vi "error_channelIndex.vi"() -> (0 "error out":errorcluster)   [LabVIEW 2020, in "NI_ExcelFile.lvlib"]
uses:
  <vilib>/express/express shared/NI_ExcelFile/NI_ExcelFile.lvlib
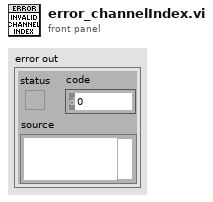
[diagram p1: front panel]
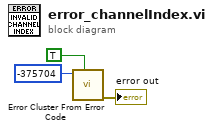
[diagram p0: block diagram]
diagram:
  n1 = call <vilib>:"Error Cluster From Error Code.vi"("show call chain? (False)"=TRUE, "error code (0)"=-375704 ("code")) -> ("error out"=→"error out":errorcluster)  [unwired: 7 in]
